vi "rtWrite.vi"(0 "File":refnum<k34>, 5 "Timestamp":timestamp, 7 "OnBottom":bool, 9 "Input Array":dbl[](array[numeric]), 11 "error in":errorcluster) -> (4 "File out":refnum<k34>, 15 "error out":errorcluster)   [LabVIEW 2019]
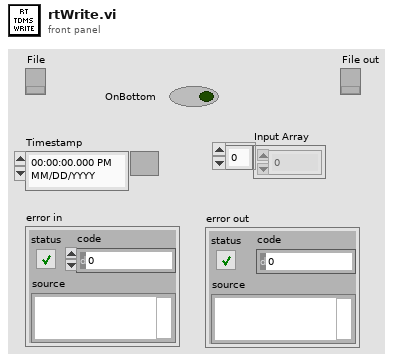
[diagram p1: front panel]
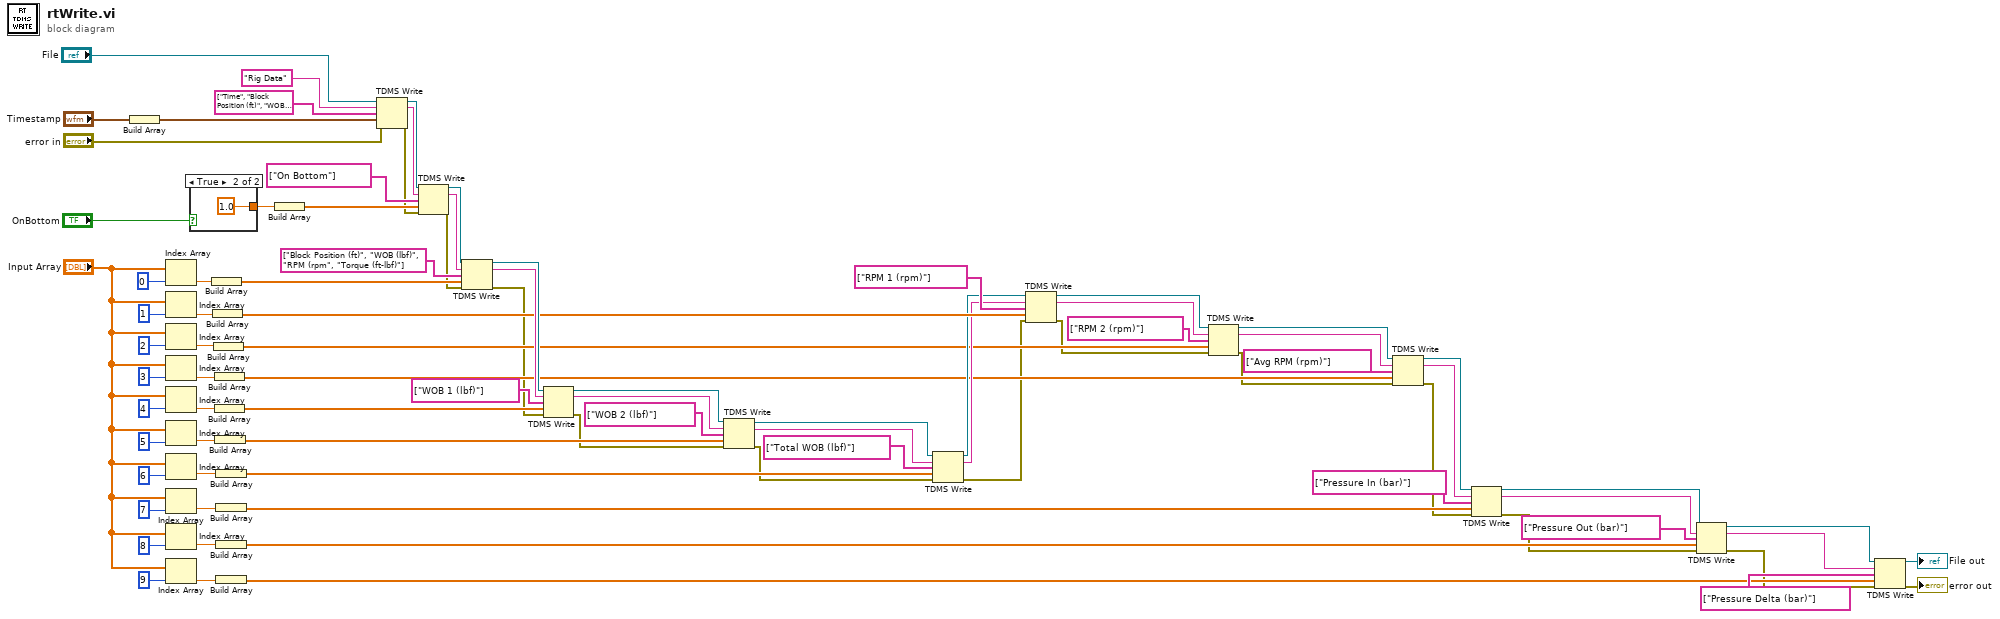
[diagram p0: block diagram]
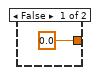
[diagram p2: hidden frame]
diagram:
  n1 = Build Array("Timestamp") -> (w73:timestamp[])
  n2 = Index Array(array="Input Array", index=0) -> (element=w66:dbl)
  n3 = Index Array(array="Input Array", index=1) -> (element=w65:dbl)
  n4 = Index Array(array="Input Array", index=2) -> (element=w64:dbl)
  n5 = Index Array(array="Input Array", index=3) -> (element=w63:dbl)
  n6 = Index Array(array="Input Array", index=4) -> (element=w62:dbl)
  n7 = Index Array(array="Input Array", index=5) -> (element=w61:dbl)
  n8 = Index Array(array="Input Array", index=6) -> (element=w60:dbl)
  n9 = Index Array(array="Input Array", index=7) -> (element=w59:dbl)
  n10 = Index Array(array="Input Array", index=8) -> (element=w58:dbl)
  n11 = Index Array(array="Input Array", index=9) -> (element=w57:dbl)
  n12 = case shown="True" "OnBottom" {
    tunnel: [0.0 1.0] -> w32
    frame False {
    }
    frame True {
    }
  }
  n13 = Build Array(w66) -> (w56:dbl[])
  n14 = Build Array(w65) -> (w42:dbl[])
  n15 = Build Array(w64) -> (w39:dbl[])
  n16 = Build Array(w63) -> (w33:dbl[])
  n17 = Build Array(w62) -> (w53:dbl[])
  n18 = Build Array(w61) -> (w50:dbl[])
  n19 = Build Array(w60) -> (w47:dbl[])
  n20 = Build Array(w59) -> (w23:dbl[])
  n21 = Build Array(w58) -> (w10:dbl[])
  n22 = Build Array(w57) -> (w9:dbl[])
  n23 = Build Array(w32) -> (w29:dbl[])
  n24 = TDMS Write(0:"File", 5:"Rig Data" ("group name in (Untitled)"), 7:string[] ["Time", "Block Position (ft)", "WOB (lbf)", "RPM (rpm)", "Torque (ft-lbf)"] ("channel name(s) in (Untitled)"), 9:w73, 11:"error in") -> (4:w25:refnum<k34>, 6:w26:string, 15:w12:errorcluster)  [unwired: 1 in, 1 out]
  n25 = TDMS Write(0:w25, 5:w26, 7:string[] ["On Bottom"] ("channel name(s) in (Untitled)"), 9:w29, 11:w12) -> (4:w27:refnum<k34>, 6:w28:string, 15:w13:errorcluster)  [unwired: 1 in, 1 out]
  n26 = TDMS Write(0:w27, 5:w28, 7:string[] ["Block Position (ft)", "WOB (lbf)", "RPM (rpm", "Torque (ft-lbf)"] ("channel name(s) in (Untitled)"), 9:w56, 11:w13) -> (4:w51:refnum<k34>, 6:w52:string, 15:w14:errorcluster)  [unwired: 1 in, 1 out]
  n27 = TDMS Write(0:w51, 5:w52, 7:string[] ["WOB 1 (lbf)"] ("channel name(s) in (Untitled)"), 9:w53, 11:w14) -> (4:w48:refnum<k34>, 6:w49:string, 15:w15:errorcluster)  [unwired: 1 in, 1 out]
  n28 = TDMS Write(0:w48, 5:w49, 7:string[] ["WOB 2 (lbf)"] ("channel name(s) in (Untitled)"), 9:w50, 11:w15) -> (4:w46:refnum<k34>, 6:w45:string, 15:w16:errorcluster)  [unwired: 1 in, 1 out]
  n29 = TDMS Write(0:w46, 5:w45, 7:string[] ["Total WOB (lbf)"] ("channel name(s) in (Untitled)"), 9:w47, 11:w16) -> (4:w41:refnum<k34>, 6:w40:string, 15:w17:errorcluster)  [unwired: 1 in, 1 out]
  n30 = TDMS Write(0:w41, 5:w40, 7:string[] ["RPM 1 (rpm)"] ("channel name(s) in (Untitled)"), 9:w42, 11:w17) -> (4:w38:refnum<k34>, 6:w37:string, 15:w18:errorcluster)  [unwired: 1 in, 1 out]
  n31 = TDMS Write(0:w38, 5:w37, 7:string[] ["RPM 2 (rpm)"] ("channel name(s) in (Untitled)"), 9:w39, 11:w18) -> (4:w35:refnum<k34>, 6:w34:string, 15:w19:errorcluster)  [unwired: 1 in, 1 out]
  n32 = TDMS Write(0:w35, 5:w34, 7:string[] ["Avg RPM (rpm)"] ("channel name(s) in (Untitled)"), 9:w33, 11:w19) -> (4:w21:refnum<k34>, 6:w22:string, 15:w20:errorcluster)  [unwired: 1 in, 1 out]
  n33 = TDMS Write(0:w21, 5:w22, 7:string[] ["Pressure In (bar)"] ("channel name(s) in (Untitled)"), 9:w23, 11:w20) -> (4:w7:refnum<k34>, 6:w8:string, 15:w6:errorcluster)  [unwired: 1 in, 1 out]
  n34 = TDMS Write(0:w7, 5:w8, 7:string[] ["Pressure Out (bar)"] ("channel name(s) in (Untitled)"), 9:w10, 11:w6) -> (4:w3:refnum<k34>, 6:w4:string, 15:w5:errorcluster)  [unwired: 1 in, 1 out]
  n35 = TDMS Write(0:w3, 5:w4, 7:string[] ["Pressure Delta (bar)"] ("channel name(s) in (Untitled)"), 9:w9, 11:w5) -> (4:→"File out":refnum<k34>, 15:→"error out":errorcluster)  [unwired: 1 in, 2 out]
